vi "2.Serrure_Numerique.vi"() -> ()   [LabVIEW 2018]
panel:
  out "Led":bool
  in  "Button 3":dbl(knob) scale=0.0..9.0
  in  "Button 2":dbl(knob) scale=0.0..9.0
  in  "Button":dbl(knob) scale=0.0..9.0
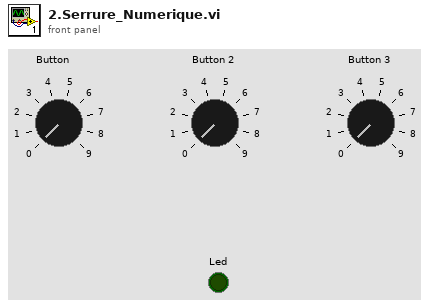
[diagram p1: front panel]
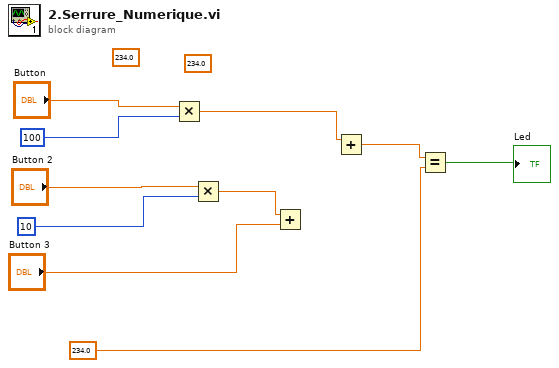
[diagram p0: block diagram]
diagram:
  (unwired) 234.0 ("Button 3")
  (unwired) 234.0 ("Button 2")
  n1 = Multiply(x="Button", y=100) -> (x*y=w6:dbl)
  n2 = Multiply(x="Button 2", y=10) -> (x*y=w4:dbl)
  n3 = Add(x=w4, y="Button 3") -> ()  [unwired: 1 out]
  n4 = Add(x=w6) -> (x+y=w2:dbl)  [unwired: 1 in]
  n5 = Equal?(x=w2, y=234.0 ("Button")) -> (x = y?=→"Led":bool)
